vi "solar_tcp Debug Get.vi"(8 "error in (no error)":errorcluster, 9 "Clear? (F)":bool, 10 "Filter Messages Only? (F)":bool, 11 "TCP Data in":T1={"Connected"=FALSE, "Config"={"TCPServer"=enum."SERVER", "ServerPort"=0, "IPAddress"="", "ClientPort"=0, "HdrSizeBytes"=4, "HdrLenSubtractBytes"=0, "HdrLenOffsetBits"=0, "HdrLenSizeBits"=32}, "Clients"=[], "ConnectionID"=refnum, "Debug"=[]} {"Debug"."Time" format="%<%Y-%m-%d\n%H:%M:%S%3u>T"}) -> (0 "error out":errorcluster, 2 "Debug Log":string, 3 "TCP Data out":T1={"Connected"=FALSE, "Config"={"TCPServer"=enum."SERVER", "ServerPort"=0, "IPAddress"="", "ClientPort"=0, "HdrSizeBytes"=4, "HdrLenSubtractBytes"=0, "HdrLenOffsetBits"=0, "HdrLenSizeBits"=32}, "Clients"=[], "ConnectionID"=refnum, "Debug"=[]} {"Debug"."Time" format="%<%Y-%m-%d\n%H:%M:%S%3u>T"})   [LabVIEW 2018]
doc: "This returns the TCP debug log string. To filter on valid messages, set <b>Filter Messages Only?</b> to true. Set <b>Clear?</b> to flush the debug messages."
uses:
  solar_tcp_ctl Config.ctl
  solar_tcp_ctl Data.ctl
  solar_tcp_ctl Action.ctl
  solar_tcp_ctl Debug.ctl
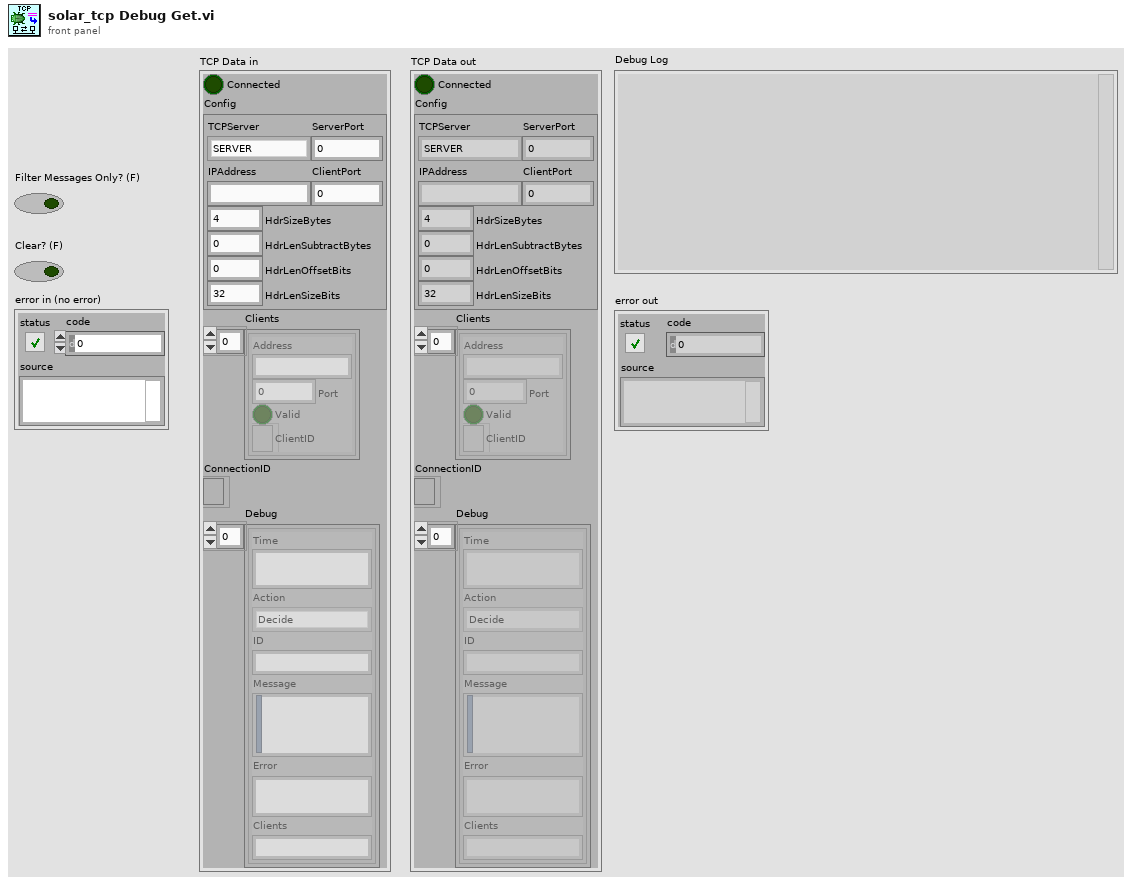
[diagram p1: front panel]
types:
  T1 = typedef "solar_tcp_ctl Data.ctl" = cluster{"Connected":bool, "Config":T2, "Clients":cluster{"Address":string, "Port":u16, "Valid":bool, "ClientID":refnum<k5>}[], "ConnectionID":refnum<k5>, "Debug":T3[]}
  T2 = typedef "solar_tcp_ctl Config.ctl" = cluster{"TCPServer":enum8{"SERVER", "CLIENT"}, "ServerPort":u16, "IPAddress":string, "ClientPort":u16, "HdrSizeBytes":i32, "HdrLenSubtractBytes":i32, "HdrLenOffsetBits":i32, "HdrLenSizeBits":i32}
  T3 = typedef "solar_tcp_ctl Debug.ctl" = cluster{"Time":timestamp, "Action":T4, "ID":string, "Message":string, "Error":string, "Clients":string}
  T4 = typedef "solar_tcp_ctl Action.ctl" = enum16{"Decide", "CreateListener", "Open", "Read", "Write", "Close", "Shutdown", "Done", "ChangePort"}
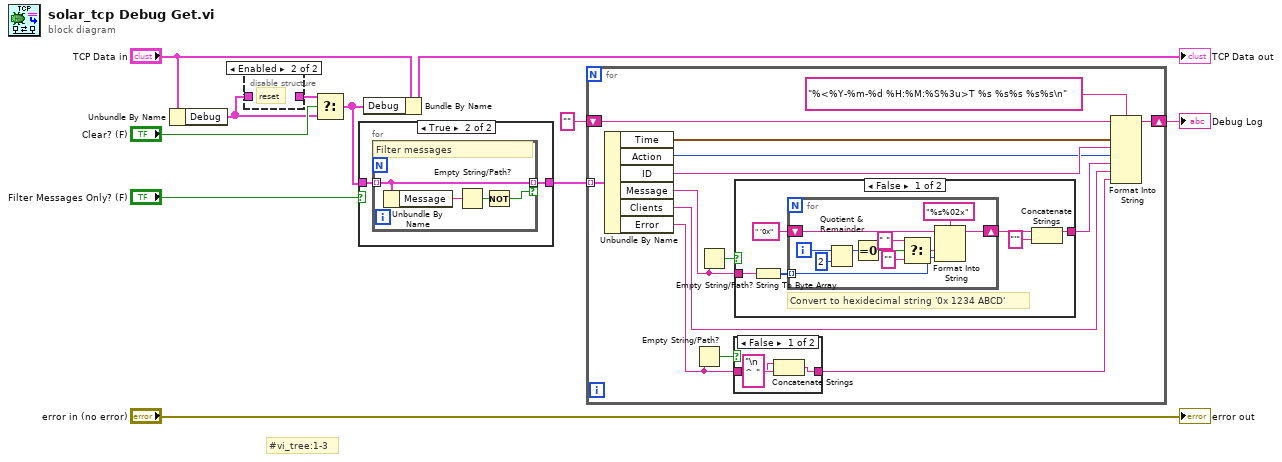
[diagram p0: block diagram]
diagram:
  # "#vi_tree:1-3"
  n1 = Unbundle By Name("TCP Data in") -> ("Debug"=w2:T3[])
  n2 = disable-structure shown="Enabled" {
    disable-tunnel: w2 -> [w12 _]
    disable-tunnel: [w12 _] -> w1
    frame Disabled {
    }
    frame Enabled {
      # "reset"
    }
  }
  n3 = Select(t=w1, s="Clear? (F)", f=w2) -> (s? t:f=w5:T3[])
  n4 = case shown="True" "Filter Messages Only? (F)" {
    tunnel: w5 -> [w13 w15]
    tunnel: [w13 w14] -> w6
    frame False {
    }
    frame True {
      n5 = for {
        tunnel: w15 -> [w18] mode=indexing
        tunnel: [w18] -> w14 mode=indexing if=w16
        # "Filter messages"
        n6 = Unbundle By Name(w18) -> ("Message"=w19:string)
        n7 = Empty String/Path?(string/path=w19) -> (empty?=w17:bool)
        n8 = Not(x=w17) -> (.not. x?=w16:bool)
      }
    }
  }
  n9 = Bundle By Name(cluster="TCP Data in", "Debug"=w5) -> (→"TCP Data out":T1)
  n10 = for {
    tunnel: w6 -> [w33] mode=indexing
    shift-right: [w31] -> w11
    shift-left: "" ("f") -> [w30]
    n11 = Unbundle By Name(w33) -> ("Time"=w29:timestamp, "Action"=w22:T4, "ID"=w23:string, "Message"=w25:string, "Clients"=w20:string, "Error"=w32:string)
    n12 = Empty String/Path?(string/path=w32) -> (empty?=w27:bool)
    n13 = Empty String/Path?(string/path=w25) -> (empty?=w26:bool)
    n14 = case shown="False" w27 {
      tunnel: w32 -> [w53 w54]
      tunnel: [w51 w54] -> w21
      frame False {
        n15 = Concatenate Strings("\n ^ " ("string"), w53) -> (w51:string)
      }
      frame True {
      }
    }
    n16 = case shown="False" w26 {
      tunnel: w25 -> [w37 _]
      tunnel: [w35 _] -> w24
      frame False {
        # "Convert to hexidecimal string '0x 1234 ABCD'"
        n17 = String To Byte Array(string=w37) -> (unsigned byte array=w39:u8[])
        n18 = for {
          tunnel: w39 -> [w40] mode=indexing
          shift-right: [w50] -> w36
          shift-left: " '0x" -> [w49]
          i -> [w47]
          n19 = Quotient & Remainder(x=w47, y=2) -> (x-y*floor(x/y)=w45:i32)  [unwired: 1 out]
          n20 = Equal To 0?(x=w45) -> (x = 0?=w44:bool)
          n21 = Select(t=" ", s=w44, f="") -> (s? t:f=w41:string)
          n22 = Format Into String(format string="%s%02x", initial string=w49, w41, w40) -> (resulting string=w50:string)  [unwired: 1 in, 1 out]
        }
        n23 = Concatenate Strings(w36, "'" ("string")) -> (w35:string)
      }
      frame True {
      }
    }
    n24 = Format Into String(format string="%<%Y-%m-%d %H:%M:%S%3u>T %s %s%s %s%s\n", initial string=w30, w29, w23, w22, w24, w20, w21) -> (resulting string=w31:string)  [unwired: 1 in, 1 out]
  }
  "Debug Log" <- w11
  "error out" <- "error in (no error)"
